vi "Write Size.vi"(8 "error in (no error)":errorcluster, 11 "Picture in":refnum<class "Picture.lvclass">) -> (0 "error out":errorcluster, 3 "Picture out":refnum<class "Picture.lvclass">)   [LabVIEW 2018, in "Picture.lvclass"]
uses:
  Picture.lvclass
  Picture.lvclass/Picture.ctl
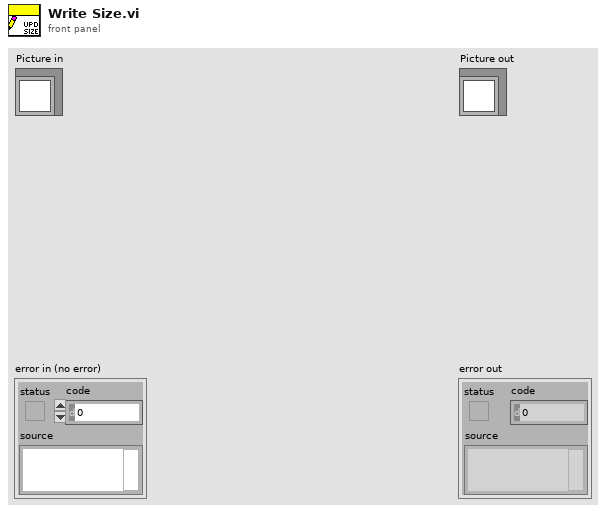
[diagram p1: front panel]
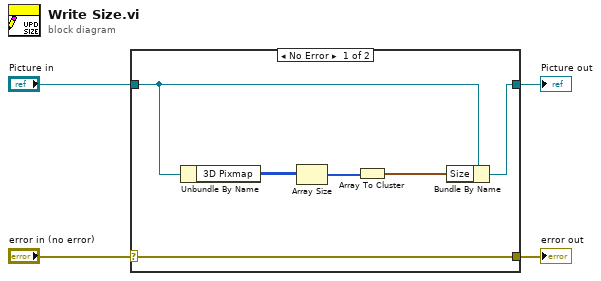
[diagram p0: block diagram]
diagram:
  n1 = case shown="No Error" "error in (no error)" {
    selector: "error in (no error)" -> [w10 w11]
    tunnel: [w10 w11] -> w3
    tunnel: [w9 w12] -> w1
    tunnel: "Picture in" -> [w6 w12]
    frame No Error {
      n2 = Unbundle By Name(w6) -> ("3D Pixmap"=w8:u32[][][])
      n3 = Array Size(array=w8) -> (size(s)=w7:i32[])
      n4 = Array To Cluster(array=w7) -> (cluster=w5:cluster{"[0]":i32, "[1]":i32, "[2]":i32})
      n5 = Bundle By Name(cluster=w6, "Size"=w5) -> (w9:refnum<class "Picture.lvclass">)
    }
    frame Error {
    }
  }
  "error out" <- w3
  "Picture out" <- w1
